vi "WSVCAP SHL Host TL I2C Write - Multiple Device - Unique Data.vi"(0 "C1 Data":u8[](array[numeric]) format="%.0x", 3 "FPGA":T1, 5 "C2 Data":u8[](array[numeric]) format="%.0x", 7 "C3 Data":u8[](array[numeric]) format="%.0x", 9 "Sub Address":u8=20 format="%.0x", 11 "error in":errorcluster, 12 "Log (T)":bool=TRUE, 13 "DUT Mask Array (All)":bool[][](array[boolean])=[[TRUE, TRUE, TRUE, TRUE, TRUE, TRUE, TRUE, TRUE, TRUE, TRUE, TRUE, TRUE, TRUE, TRUE, TRUE, TRUE, TRUE, TRUE, TRUE, TRUE, TRUE, TRUE, TRUE, TRUE, TRUE, TRUE, TRUE, TRUE, TRUE, TRUE, TRUE, TRUE, TRUE, TRUE, TRUE, TRUE], [TRUE, TRUE, TRUE, TRUE, TRUE, TRUE, TRUE, TRUE, TRUE, TRUE, TRUE, TRUE, TRUE, TRUE, TRUE, TRUE, TRUE, TRUE, TRUE, TRUE, TRUE, TRUE, TRUE, TRUE, TRUE, TRUE, TRUE, TRUE, TRUE, TRUE, TRUE, TRUE, TRUE, TRUE, TRUE, TRUE], [TRUE, TRUE, TRUE, TRUE, TRUE, TRUE, TRUE, TRUE, TRUE, TRUE, TRUE, TRUE, TRUE, TRUE, TRUE, TRUE, TRUE, TRUE, TRUE, TRUE, TRUE, TRUE, TRUE, TRUE, TRUE, TRUE, TRUE, TRUE, TRUE, TRUE, TRUE, TRUE, TRUE, TRUE, TRUE, TRUE], [FALSE, FALSE, FALSE, FALSE, FALSE, FALSE, FALSE, FALSE, FALSE, FALSE, FALSE, FALSE, FALSE, FALSE, FALSE, FALSE, TRUE, FALSE, FALSE, FALSE, FALSE, FALSE, TRUE, FALSE, FALSE, FALSE, FALSE, FALSE, FALSE, FALSE, FALSE, TRUE, FALSE, FALSE, FALSE, FALSE]], 14 "DUT Mask Mode (All)":T2=enum."All") -> (15 "error out":errorcluster)   [LabVIEW 2012]
uses:
  Type Defs/WSVCAP SHL I2C DUT Mask Mode Enum.ctl
  Type Defs/WSVCAP SHL I2C FPGA Enum.ctl
panel:
  out "C3 Data Out":u8[](array[numeric]) format="%.0x"
  out "Socket Mask Set [U64]":u64[](array[numeric]) format="%012x"
  out "C2 Data Out":u8[](array[numeric]) format="%.0x"
  out "C1 Data Out":u8[](array[numeric]) format="%.0x"
  # "DUT 01"
  # "DUT 02"
  # "DUT 03"
  # "DUT 04"
  # "DUT 05"
  # "DUT 06"
  # "DUT 07"
  # "DUT 08"
  # "DUT 09"
  # "DUT 10"
  # "DUT 11"
  # "DUT 12"
  # "DUT 13"
  # "DUT 14"
  # "DUT 15"
  # "DUT 16"
  # "DUT 17"
  # "DUT 18"
  # "DUT 19"
  # "DUT 20"
  # "DUT 21"
  # "DUT 22"
  # "DUT 23"
  # "DUT 24"
  # "DUT 25"
  # "DUT 26"
  # "DUT 27"
  # "DUT 28"
  # "DUT 29"
  # "DUT 30"
  # "DUT 31"
  # "DUT 32"
  # "DUT 33"
  # "DUT 34"
  # "DUT 35"
  # "DUT 36"
  # "C1"
  # "C2"
  # "C3"
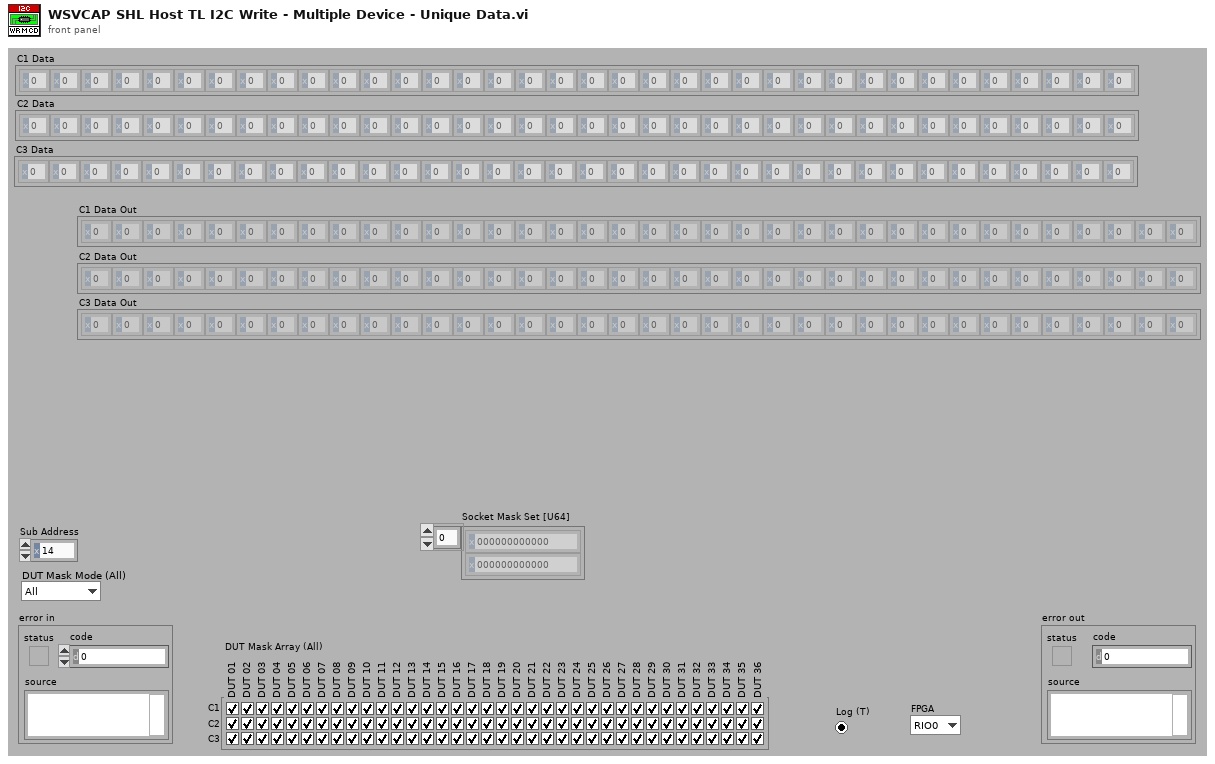
[diagram p1: front panel]
types:
  T1 = typedef "WSVCAP SHL I2C FPGA Enum.ctl" = enum16{"RIO0", "RIO1"}
  T2 = typedef "WSVCAP SHL I2C DUT Mask Mode Enum.ctl" = enum16{"Custom", "C1", "C2", "C3", "All"}
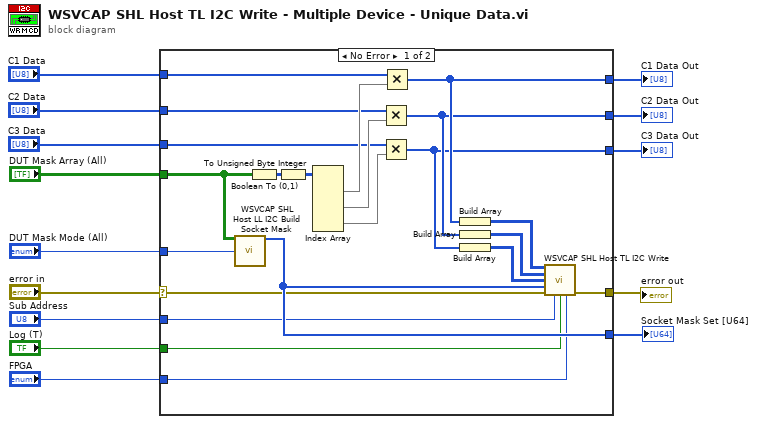
[diagram p0: block diagram]
diagram:
  n1 = case shown="No Error" "error in" {
    selector: "error in" -> [w26 w37]
    tunnel: [w36 w37] -> w14
    tunnel: "Sub Address" -> [w22 _]
    tunnel: [w27 _] -> w11
    tunnel: [w28 _] -> w10
    tunnel: [w33 _] -> w9
    tunnel: "DUT Mask Array (All)" -> [w20 _]
    tunnel: "Log (T)" -> [w25 _]
    tunnel: [w21 _] -> w6
    tunnel: "DUT Mask Mode (All)" -> [w19 _]
    tunnel: "C1 Data" -> [w18 _]
    tunnel: "C2 Data" -> [w17 _]
    tunnel: "C3 Data" -> [w16 _]
    tunnel: "FPGA" -> [w15 _]
    frame No Error {
      n2 = call "WSVCAP SHL Host LL I2C Build Socket Mask.vi"("DUT Mask Array"=w20, "DUT Mask Mode (Custom)"=w19) -> ("Socket Mask Set [U64]"=w33:u64[])  [unwired: 13 in]
      n3 = Boolean To (0,1)(Boolean=w20) -> (0, 1=w32:i16[][])
      n4 = To Unsigned Byte Integer(number=w32) -> (unsigned 8bit integer=w29:u8[][])
      n5 = Index Array(array=w29) -> (element #1=w31:u8[], element #2=w30:u8[], element #3=w24:u8[])  [unwired: 6 in]
      n6 = Multiply(x=w17, y=w30) -> (x*y=w27:u8[])
      n7 = Multiply(x=w16, y=w24) -> (x*y=w21:u8[])
      n8 = Multiply(x=w18, y=w31) -> (x*y=w28:u8[])
      n9 = Build Array(w28) -> (w35:u8[][])
      n10 = Build Array(w27) -> (w34:u8[][])
      n11 = Build Array(w21) -> (w23:u8[][])
      n12 = call "WSVCAP SHL Host TL I2C Write.vi"("C1 Data Out"=w35, "C2 Data Out"=w34, "C3 Data Out"=w23, "Socket Mask Set [U64]"=w33, "error in"=w26, "Sub Address"=w22, "Log (T)"=w25, "FPGA"=w15) -> ("error out"=w36:errorcluster)  [unwired: 7 in]
    }
    frame Error {
    }
  }
  "error out" <- w14
  "C1 Data Out" <- w10
  "C2 Data Out" <- w11
  "Socket Mask Set [U64]" <- w9
  "C3 Data Out" <- w6
